vi "Link Receive Parameters.vi"(7 "Parameter W Table in":refnum<class "Registry.lvclass">, 8 "error in (no error)":errorcluster, 11 "Message in":refnum<class "Message.lvclass">) -> (0 "error out":errorcluster, 5 "Parameter W Table out":refnum<class "Registry.lvclass">)   [LabVIEW 2020, in "BCI-1553 API.lvlib" / "Message.lvclass"]
doc: "<DO NOT CALL>\n\nIf this is a receive message, we take all the parameters and add them to the parameter write table."
uses:
  Message.lvclass
  Dependencies/Registry/Registry.lvclass
  TypeDefs/Command Type.ctl
  Message.lvclass/Message.ctl
  Dependencies/Registry/Registry.lvclass/Registry.ctl
  BCI-1553 API.lvlib
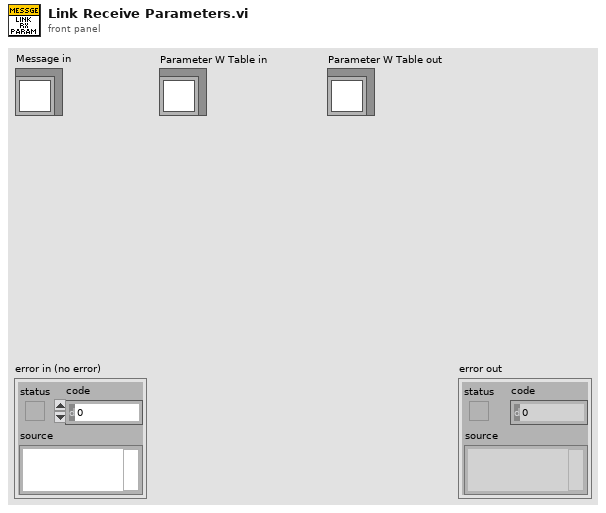
[diagram p1: front panel]
types:
  T1 = typedef "BCI-1553 API.lvlib/Command Type.ctl" = enum16{"Transmit", "Receive"}
  T2 = typedef "BCI-1553 API.lvlib/Parameter Table Data.ctl" = cluster{"Parameter Name":string, "Base Word":u16, "Address":u16, "Value":u64, "Mask":u16[], "Scaling Info":T3}
  T3 = typedef "BCI-1553 API.lvlib/Scaling Information.ctl" = cluster{"Bit Offset":i32, "Bit Count":i32, "LSB Resolution":dbl, "2's Complement":bool, "Big Endian":bool, "Sign Bit":bool}
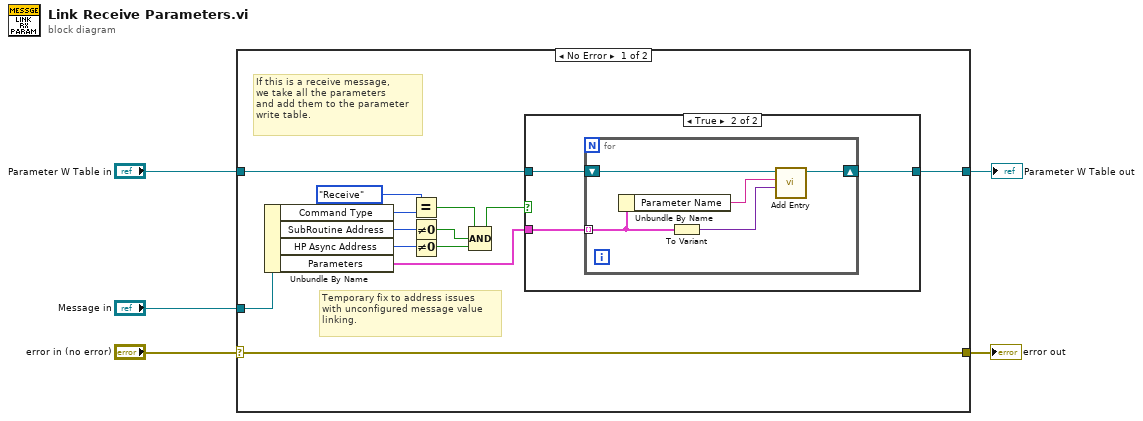
[diagram p0: block diagram]
diagram:
  n1 = case shown="No Error" "error in (no error)" {
    selector: "error in (no error)" -> [w18 w29]
    tunnel: [w18 w29] -> w4
    tunnel: "Message in" -> [w15 _]
    tunnel: "Parameter W Table in" -> [w17 w28]
    tunnel: [w16 w28] -> w1
    frame No Error {
      # "Temporary fix to address issues\nwith unconfigured message value\nlinking."
      # "If this is a receive message,\nwe take all the parameters\nand add them to the parameter\nwrite table."
      n2 = Unbundle By Name(w15) -> ("Command Type"=w14:T1, "SubRoutine Address"=w9:u16, "HP Async Address"=w8:u16, "Parameters"=w13:T2[])
      n3 = Equal?(x=Command_Type."Receive", y=w14) -> (x = y?=w7:bool)
      n4 = Not Equal To 0?(x=w9) -> (x != 0?=w10:bool)
      n5 = Not Equal To 0?(x=w8) -> (x != 0?=w11:bool)
      n6 = Compound Arithmetic op=AND(w7, w10, w11) -> (w6:bool)
      n7 = case shown="True" w6 {
        tunnel: w17 -> [w19 w22]
        tunnel: [w19 w21] -> w16
        tunnel: w13 -> [_ w20]
        frame False {
        }
        frame True {
          n8 = for {
            shift-right: [w26] -> w21
            shift-left: w22 -> [w27]
            tunnel: w20 -> [w25] mode=indexing
            n9 = Unbundle By Name(w25) -> ("Parameter Name"=w23:string)
            n10 = To Variant(anything=w25) -> (Variant=w24:variant)
            n11 = call "Add Entry.vi"("Value"=w24, "Key"=w23, "Registry in"=w27) -> ("Registry out"=w26:refnum<class "Registry.lvclass">)  [unwired: 6 in, 2 out]
          }
        }
      }
    }
    frame Error {
    }
  }
  "error out" <- w4
  "Parameter W Table out" <- w1
